vi "Run Command Gavin idk.vi"(2 "Line Index In":i32, 3 "Script":string) -> (0 "Line Index Out":i32, 1 "Done":bool)   [LabVIEW 2017, in "Apple script.lvlib"]
doc: "Looks at a line and runs the appropriate command. Add new commands to this vi."
uses:
  Apple script.lvlib
  Robot Global Data.vi
  <vilib>/addons/control/pid/pid.llb/PID.vi
  <vilib>/addons/control/pid/pid.llb/PID (DBL).vi
  Angle Distance.vi
  Pigeon Gyro.vi
  Encoders.vi
  Swerve Goto.vi
  <vilib>/Rock Robotics/Network Tables/NT Write Value.vi
  <vilib>/Rock Robotics/Network Tables/NT Write Numeric Array.vi
  Parse Number.vi
  Timer.vi
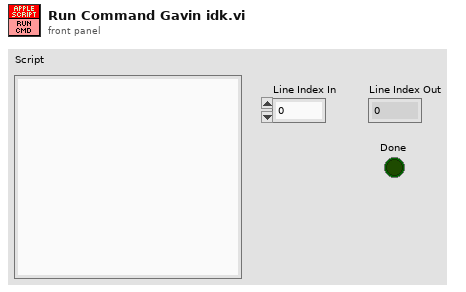
[diagram p1: front panel]
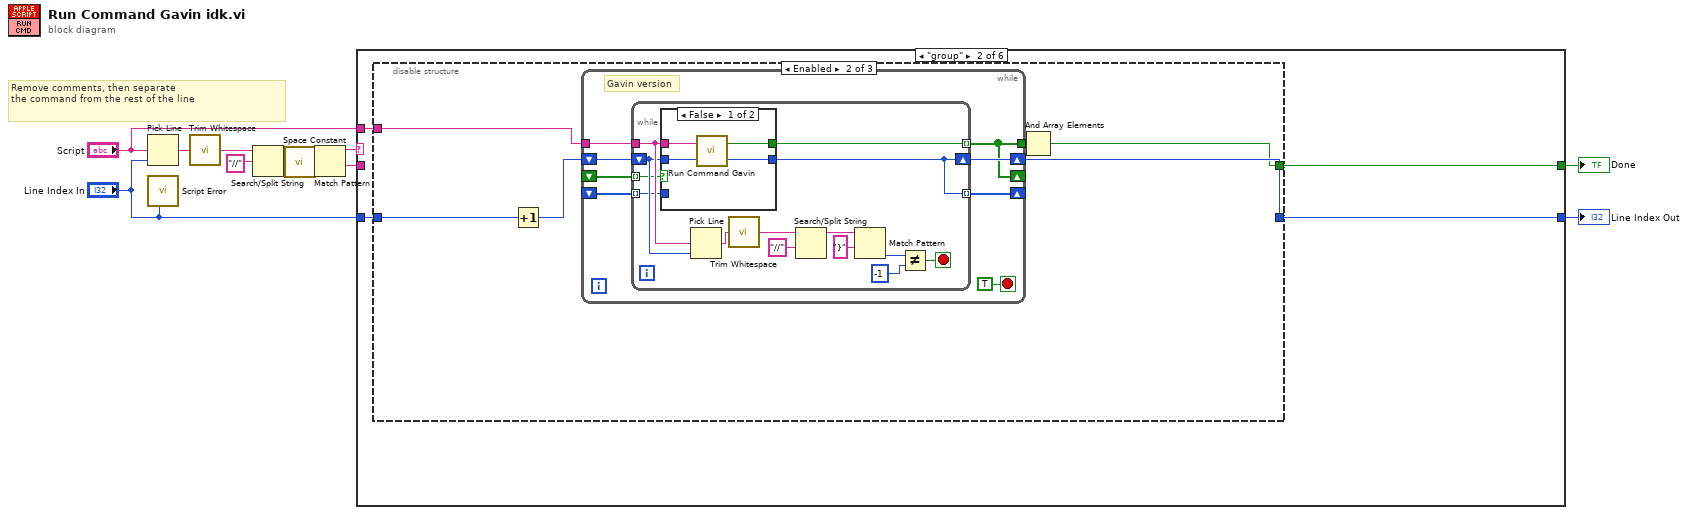
[diagram p0: block diagram]
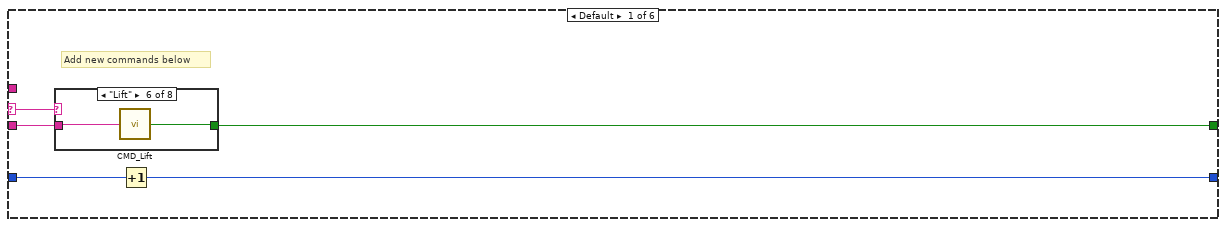
[diagram p2: hidden frame]
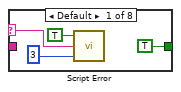
[diagram p3: hidden frame]
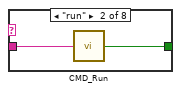
[diagram p4: hidden frame]
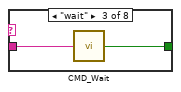
[diagram p5: hidden frame]
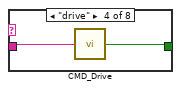
[diagram p6: hidden frame]
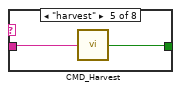
[diagram p7: hidden frame]
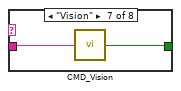
[diagram p8: hidden frame]
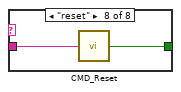
[diagram p9: hidden frame]
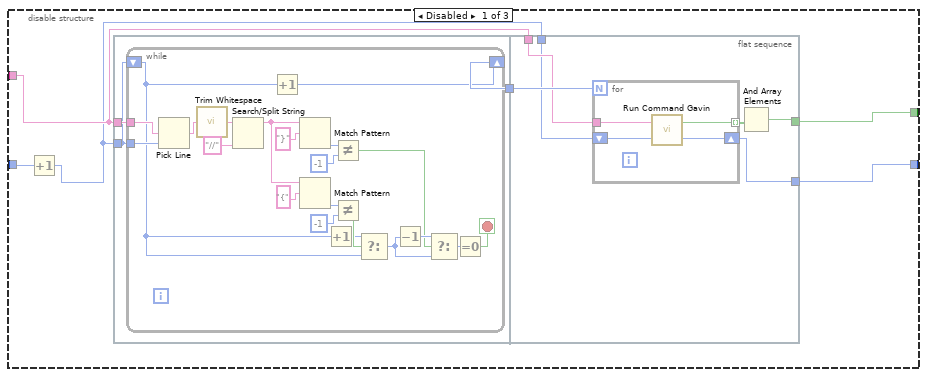
[diagram p10: hidden frame]
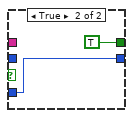
[diagram p11: hidden frame]
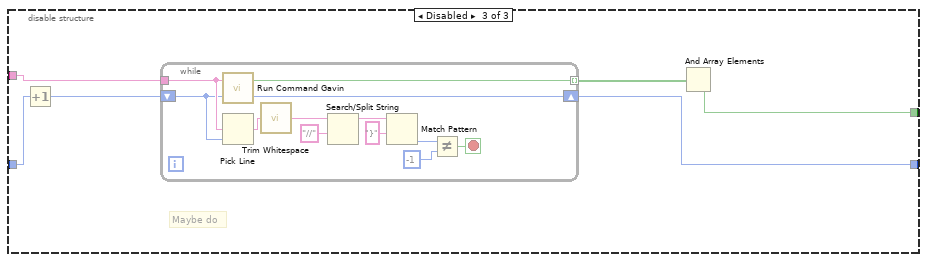
[diagram p12: hidden frame]
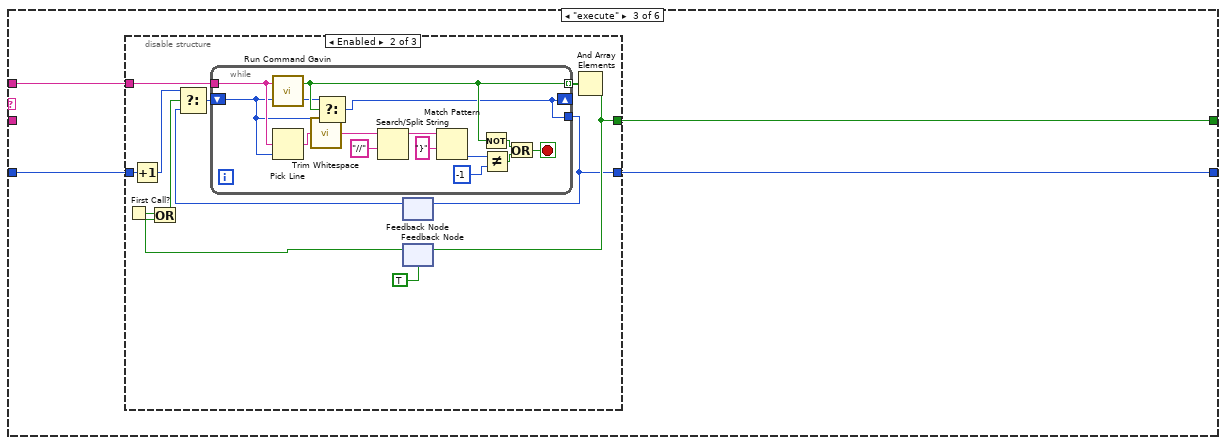
[diagram p13: hidden frame]
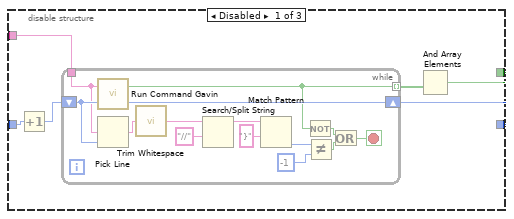
[diagram p14: hidden frame]
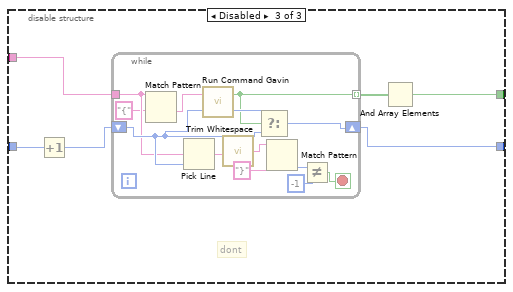
[diagram p15: hidden frame]
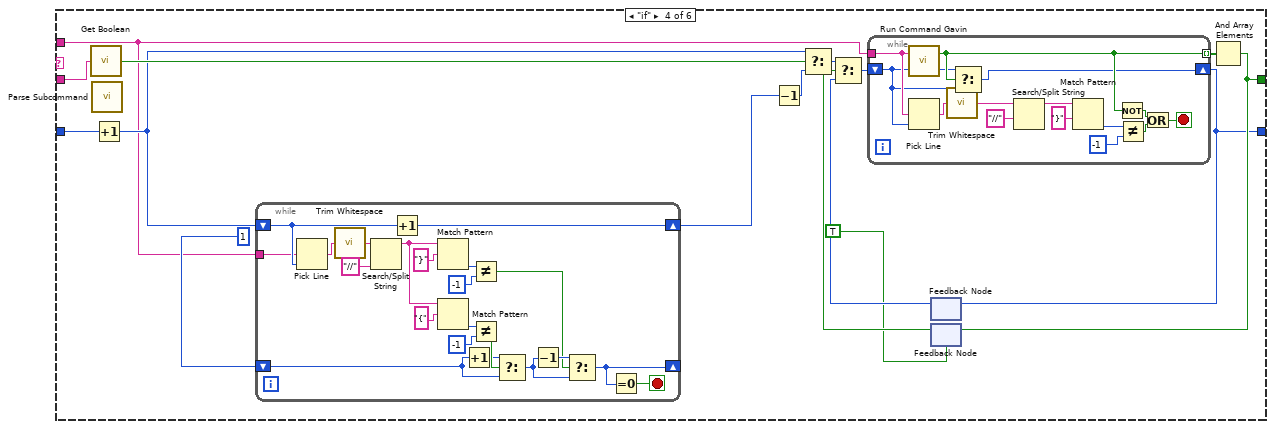
[diagram p16: hidden frame]
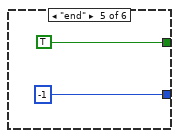
[diagram p17: hidden frame]
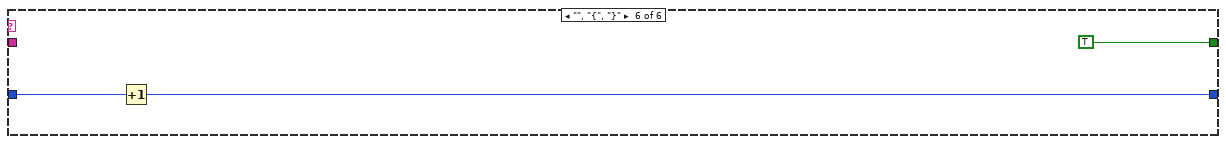
[diagram p18: hidden frame]
diagram:
  # "Remove comments, then separate\nthe command from the rest of the line"
  n1 = Pick Line(multi-line string="Script", line index="Line Index In") -> (output string=w8:string)  [unwired: 1 in]
  n2 = call "Script Error.vi"("Line Number"="Line Index In") -> ()  [unwired: 4 in, 1 out]
  n3 = call <vilib>:"Trim Whitespace.vi"("string"=w8) -> ("trimmed string"=w6:string)  [unwired: 1 in]
  n4 = Search/Split String(string=w6, search string/char (-)="//") -> (substring before match=w5:string)  [unwired: 1 in, 2 out]
  n5 = call <vilib>:"Space Constant.vi"() -> ("String"=w11:string)
  n6 = Match Pattern(string=w5, regular expression=w11) -> (before substring=w4:string, after substring=w3:string)  [unwired: 1 in, 2 out]
  n7 = case shown="\"group\"" w4 {
    selector: w4 -> [w14 _ _ _ _ _]
    tunnel: "Script" -> [_ w38 w131 w203 _ _]
    tunnel: "Line Index In" -> [w16 w36 w132 w215 _ w256]
    tunnel: [w13 w35 w134 w216 TRUE ("Running") TRUE ("Running")] -> w2
    tunnel: [w15 w37 w133 w213 -1 ("Line Index Out") w255] -> w1
    tunnel: w3 -> [w12 _ _ w214 _ _]
    frame Default {
      # "Add new commands below"
      n8 = case shown="\"Lift\"" w14 {
        selector: w14 -> [w17 _ _ _ _ _ _ _]
        tunnel: [TRUE w21 w24 w25 w27 w29 w31 w33] -> w13
        tunnel: w12 -> [_ w22 w23 w26 w28 w30 w32 w34]
        frame Default {
          n9 = call "Script Error.vi"("Error?"=TRUE, "Error Details"=w17, "Error Code"=3) -> ()  [unwired: 2 in, 1 out]
        }
        frame "run" {
          n10 = call "CMD_Run.vi"("Line"=w22) -> ("Done"=w21:bool)
        }
        frame "wait" {
          n11 = call "CMD_Wait.vi"("Line"=w23) -> ("Done"=w24:bool)
        }
        frame "drive" {
          n12 = call "CMD_Drive.vi"("Line"=w26) -> ("Done"=w25:bool)
        }
        frame "harvest" {
          n13 = call "CMD_Harvest.vi"("Line"=w28) -> ("Done"=w27:bool)
        }
        frame "Lift" {
          n14 = call "CMD_Lift.vi"("Line"=w30) -> ("Done"=w29:bool)
        }
        frame "Vision" {
          n15 = call "CMD_Vision.vi"("Line"=w32) -> ("Done"=w31:bool)
        }
        frame "reset" {
          n16 = call "CMD_Reset.vi"("Line"=w34) -> ("Done"=w33:bool)
        }
      }
      n17 = Increment(x=w16) -> (x+1=w15:i32)
    }
    frame "group" {
      n18 = disable-structure shown="Enabled" {
        disable-tunnel: w38 -> [w40 w82 w118]
        disable-tunnel: [w43 w80 w115] -> w37
        disable-tunnel: w36 -> [w42 w81 w117]
        disable-tunnel: [w44 w79 w113] -> w35
        frame Disabled {
          n19 = Increment(x=w42) -> (x+1=w39:i32)
          n20 = flat-sequence {
            tunnel: w40 -> [w46]
            tunnel: [w47] -> w41
            tunnel: w39 -> [w45]
            tunnel: [w74] -> w44
            tunnel: [w73] -> w43
            tunnel: w41 -> [w72]
            tunnel: w40 -> [w70]
            tunnel: w39 -> [w69]
            frame #0 {
              n21 = while {
                shift-right: [w68] -> w47
                shift-left: w45 -> [w48]
                tunnel: w46 -> [w51]
                tunnel: w45 -> [w50]
                stop <- w49 stop-if-true
                n22 = Pick Line(multi-line string=w51, line index=w50) -> (output string=w64:string)  [unwired: 1 in]
                n23 = call <vilib>:"Trim Whitespace.vi"("string"=w64) -> ("trimmed string"=w65:string)  [unwired: 1 in]
                n24 = Search/Split String(string=w65, search string/char (-)="//") -> (substring before match=w58:string)  [unwired: 1 in, 2 out]
                n25 = Increment(x=w48) -> (x+1=w68:i32)
                n26 = Match Pattern(string=w58, regular expression="}" ("search string/char (-)")) -> (offset past match=w67:i32)  [unwired: 1 in, 3 out]
                n27 = Match Pattern(string=w58, regular expression="{" ("search string/char (-)")) -> (offset past match=w59:i32)  [unwired: 1 in, 3 out]
                n28 = Increment(x=w48) -> (x+1=w56:i32)
                n29 = Not Equal?(x=w67, y=-1) -> (x != y?=w53:bool)
                n30 = Not Equal?(x=w59, y=-1) -> (x != y?=w57:bool)
                n31 = Select(t=w56, s=w57, f=w48) -> (s? t:f=w54:i32)
                n32 = Decrement(x=w54) -> (x-1=w55:i32)
                n33 = Select(t=w55, s=w53, f=w54) -> (s? t:f=w52:i32)
                n34 = Equal To 0?(x=w52) -> (x = 0?=w49:bool)
              }
            }
            frame #1 {
              n35 = for {
                N: w72 -> [_]
                tunnel: w70 -> [w78]
                tunnel: [w77] -> w71 mode=indexing
                shift-right: [w75] -> w73
                shift-left: w69 -> [w76]
                n36 = call "Run Command Gavin.vi"("Line Index In"=w76, "Script"=w78) -> ("Line Index Out"=w75:i32, "Done"=w77:bool)
              }
              n37 = And Array Elements(Boolean array=w71) -> (logical AND=w74:bool)
            }
          }
        }
        frame Enabled {
          n38 = Increment(x=w81) -> (x+1=w83:i32)
          n39 = while {
            tunnel: [w87] -> w84
            tunnel: w82 -> [w91]
            shift-right: [w90] -> w80
            shift-left: w83 -> [w92]
            shift-right: [w88] -> _
            shift-left: _ -> [w86]
            shift-right: [w87] -> _
            shift-left: _ -> [w85]
            stop <- TRUE stop-if-true
            # "Gavin version"
            n40 = while {
              tunnel: w91 -> [w106]
              tunnel: [w99] -> w87 mode=indexing
              shift-right: [w94] -> w90
              shift-left: w92 -> [w98]
              tunnel: w85 -> [w95] mode=indexing
              tunnel: [w94] -> w88 mode=indexing
              tunnel: w86 -> [w93] mode=indexing
              stop <- w96 stop-if-true
              n41 = case shown="False" w95 {
                tunnel: w106 -> [w110 _]
                tunnel: [w107 TRUE ("Done")] -> w99
                tunnel: w98 -> [w109 _]
                tunnel: [w108 w111] -> w94
                tunnel: w93 -> [_ w111]
                frame False {
                  n42 = call "Run Command Gavin.vi"("Line Index In"=w109, "Script"=w110) -> ("Line Index Out"=w108:i32, "Done"=w107:bool)
                }
                frame True {
                }
              }
              n43 = Pick Line(multi-line string=w106, line index=w98) -> (output string=w101:string)  [unwired: 1 in]
              n44 = call <vilib>:"Trim Whitespace.vi"("string"=w101) -> ("trimmed string"=w102:string)  [unwired: 1 in]
              n45 = Search/Split String(string=w102, search string/char (-)="//") -> (substring before match=w97:string)  [unwired: 1 in, 2 out]
              n46 = Match Pattern(string=w97, regular expression="}" ("search string/char (-)")) -> (offset past match=w104:i32)  [unwired: 1 in, 3 out]
              n47 = Not Equal?(x=w104, y=-1) -> (x != y?=w96:bool)
            }
          }
          n48 = And Array Elements(Boolean array=w84) -> (logical AND=w79:bool)
        }
        frame Disabled {
          # "Maybe do"
          n49 = Increment(x=w117) -> (x+1=w116:i32)
          n50 = while {
            tunnel: w118 -> [w130]
            tunnel: [w123] -> w114 mode=indexing
            shift-right: [w120] -> w115
            shift-left: w116 -> [w122]
            stop <- w121 stop-if-true
            n51 = call "Run Command Gavin.vi"("Line Index In"=w122, "Script"=w130) -> ("Line Index Out"=w120:i32, "Done"=w123:bool)
            n52 = Pick Line(multi-line string=w130, line index=w122) -> (output string=w125:string)  [unwired: 1 in]
            n53 = call <vilib>:"Trim Whitespace.vi"("string"=w125) -> ("trimmed string"=w126:string)  [unwired: 1 in]
            n54 = Search/Split String(string=w126, search string/char (-)="//") -> (substring before match=w119:string)  [unwired: 1 in, 2 out]
            n55 = Match Pattern(string=w119, regular expression="}" ("search string/char (-)")) -> (offset past match=w128:i32)  [unwired: 1 in, 3 out]
            n56 = Not Equal?(x=w128, y=-1) -> (x != y?=w121:bool)
          }
          n57 = And Array Elements(Boolean array=w114) -> (logical AND=w113:bool)
        }
      }
    }
    frame "execute" {
      n58 = disable-structure shown="Enabled" {
        disable-tunnel: [w137 w159 w183] -> w134
        disable-tunnel: [w138 w155 w182] -> w133
        disable-tunnel: w132 -> [w136 w166 w186]
        disable-tunnel: w131 -> [w139 w164 w187]
        frame Disabled {
          n59 = Increment(x=w136) -> (x+1=w135:i32)
          n60 = while {
            tunnel: w139 -> [w146]
            tunnel: [w142] -> w140 mode=indexing
            shift-right: [w154] -> w138
            shift-left: w135 -> [w147]
            stop <- w145 stop-if-true
            n61 = call "Run Command Gavin.vi"("Line Index In"=w147, "Script"=w146) -> ("Line Index Out"=w154:i32, "Done"=w142:bool)
            n62 = Pick Line(multi-line string=w146, line index=w147) -> (output string=w149:string)  [unwired: 1 in]
            n63 = call <vilib>:"Trim Whitespace.vi"("string"=w149) -> ("trimmed string"=w150:string)  [unwired: 1 in]
            n64 = Search/Split String(string=w150, search string/char (-)="//") -> (substring before match=w141:string)  [unwired: 1 in, 2 out]
            n65 = Match Pattern(string=w141, regular expression="}" ("search string/char (-)")) -> (offset past match=w152:i32)  [unwired: 1 in, 3 out]
            n66 = Not(x=w142) -> (.not. x?=w143:bool)
            n67 = Not Equal?(x=w152, y=-1) -> (x != y?=w144:bool)
            n68 = Or(x=w143, y=w144) -> (x .or. y?=w145:bool)
          }
          n69 = And Array Elements(Boolean array=w140) -> (logical AND=w137:bool)
        }
        frame Enabled {
          n70 = First Call?() -> (First Call?: T/F=w156:bool)
          n71 = Increment(x=w166) -> (x+1=w162:i32)
          n72 = feedback #1() -> (w161:i32)  [unwired: 1 in]
          n73 = feedback #2(TRUE) -> (w160:bool)
          n74 = Or(x=w156, y=w160) -> (x .or. y?=w157:bool)
          n75 = Select(t=w162, s=w157, f=w161) -> (s? t:f=w163:i32)
          n76 = while {
            tunnel: w164 -> [w181]
            tunnel: [w171] -> w165 mode=indexing
            shift-right: [w167] -> _
            shift-left: w163 -> [w169]
            tunnel: [w167] -> w155
            stop <- w180 stop-if-true
            n77 = call "Run Command Gavin.vi"("Line Index In"=w169, "Script"=w181) -> ("Line Index Out"=w170:i32, "Done"=w171:bool)
            n78 = Pick Line(multi-line string=w181, line index=w169) -> (output string=w175:string)  [unwired: 1 in]
            n79 = call <vilib>:"Trim Whitespace.vi"("string"=w175) -> ("trimmed string"=w176:string)  [unwired: 1 in]
            n80 = Select(t=w170, s=w171, f=w169) -> (s? t:f=w167:i32)
            n81 = Search/Split String(string=w176, search string/char (-)="//") -> (substring before match=w168:string)  [unwired: 1 in, 2 out]
            n82 = Match Pattern(string=w168, regular expression="}" ("search string/char (-)")) -> (offset past match=w178:i32)  [unwired: 1 in, 3 out]
            n83 = Not(x=w171) -> (.not. x?=w172:bool)
            n84 = Not Equal?(x=w178, y=-1) -> (x != y?=w173:bool)
            n85 = Or(x=w172, y=w173) -> (x .or. y?=w180:bool)
          }
          n86 = feedback-in #1(w155) -> ()
          n87 = And Array Elements(Boolean array=w165) -> (logical AND=w159:bool)
          n88 = feedback-in #2(w159) -> ()
        }
        frame Disabled {
          # "dont"
          n89 = Increment(x=w186) -> (x+1=w185:i32)
          n90 = while {
            tunnel: w187 -> [w190]
            tunnel: [w199] -> w184 mode=indexing
            shift-right: [w198] -> w182
            shift-left: w185 -> [w191]
            stop <- w192 stop-if-true
            n91 = Match Pattern(string=w190, regular expression="{") -> (after substring=w188:string)  [unwired: 1 in, 3 out]
            n92 = Pick Line(multi-line string=w190, line index=w191) -> (output string=w197:string)  [unwired: 1 in]
            n93 = call "Run Command Gavin.vi"("Line Index In"=w191, "Script"=w188) -> ("Line Index Out"=w200:i32, "Done"=w199:bool)
            n94 = call <vilib>:"Trim Whitespace.vi"("string"=w197) -> ("trimmed string"=w196:string)  [unwired: 1 in]
            n95 = Select(t=w200, s=w199, f=w191) -> (s? t:f=w198:i32)
            n96 = Match Pattern(string=w196, regular expression="}") -> (offset past match=w194:i32)  [unwired: 1 in, 3 out]
            n97 = Not Equal?(x=w194, y=-1) -> (x != y?=w192:bool)
          }
          n98 = And Array Elements(Boolean array=w184) -> (logical AND=w183:bool)
        }
      }
    }
    frame "if" {
      n99 = call "Get Boolean.vi"("Name"=w214) -> ("Value"=w207:bool)
      n100 = call "Parse Subcommand.vi"() -> ()  [unwired: 9 in, 7 out]
      n101 = Increment(x=w215) -> (x+1=w205:i32)
      n102 = while {
        shift-right: [w230] -> w204
        shift-left: w205 -> [w232]
        shift-right: [w218] -> _
        shift-left: 1 -> [w223]
        tunnel: w203 -> [w217]
        stop <- w219 stop-if-true
        n103 = Pick Line(multi-line string=w217, line index=w232) -> (output string=w234:string)  [unwired: 1 in]
        n104 = call <vilib>:"Trim Whitespace.vi"("string"=w234) -> ("trimmed string"=w235:string)  [unwired: 1 in]
        n105 = Search/Split String(string=w235, search string/char (-)="//") -> (substring before match=w226:string)  [unwired: 1 in, 2 out]
        n106 = Increment(x=w232) -> (x+1=w230:i32)
        n107 = Match Pattern(string=w226, regular expression="}" ("search string/char (-)")) -> (offset past match=w237:i32)  [unwired: 1 in, 3 out]
        n108 = Match Pattern(string=w226, regular expression="{" ("search string/char (-)")) -> (offset past match=w227:i32)  [unwired: 1 in, 3 out]
        n109 = Increment(x=w223) -> (x+1=w224:i32)
        n110 = Not Equal?(x=w237, y=-1) -> (x != y?=w220:bool)
        n111 = Not Equal?(x=w227, y=-1) -> (x != y?=w225:bool)
        n112 = Select(t=w224, s=w225, f=w223) -> (s? t:f=w221:i32)
        n113 = Decrement(x=w221) -> (x-1=w222:i32)
        n114 = Select(t=w222, s=w220, f=w221) -> (s? t:f=w218:i32)
        n115 = Equal To 0?(x=w218) -> (x = 0?=w219:bool)
      }
      n116 = Decrement(x=w204) -> (x-1=w201:i32)
      n117 = Select(t=w205, s=w207, f=w201) -> (s? t:f=w208:i32)
      n118 = feedback #3() -> (w209:i32)  [unwired: 1 in]
      n119 = feedback #4(TRUE) -> (w212:bool)
      n120 = Select(t=w208, s=w212, f=w209) -> (s? t:f=w211:i32)
      n121 = while {
        tunnel: w203 -> [w252]
        tunnel: [w242] -> w210 mode=indexing
        shift-right: [w239] -> w213
        shift-left: w211 -> [w240]
        stop <- w251 stop-if-true
        n122 = call "Run Command Gavin.vi"("Line Index In"=w240, "Script"=w252) -> ("Line Index Out"=w241:i32, "Done"=w242:bool)
        n123 = Pick Line(multi-line string=w252, line index=w240) -> (output string=w246:string)  [unwired: 1 in]
        n124 = call <vilib>:"Trim Whitespace.vi"("string"=w246) -> ("trimmed string"=w247:string)  [unwired: 1 in]
        n125 = Select(t=w241, s=w242, f=w240) -> (s? t:f=w239:i32)
        n126 = Search/Split String(string=w247, search string/char (-)="//") -> (substring before match=w238:string)  [unwired: 1 in, 2 out]
        n127 = Match Pattern(string=w238, regular expression="}" ("search string/char (-)")) -> (offset past match=w249:i32)  [unwired: 1 in, 3 out]
        n128 = Not(x=w242) -> (.not. x?=w243:bool)
        n129 = Not Equal?(x=w249, y=-1) -> (x != y?=w244:bool)
        n130 = Or(x=w243, y=w244) -> (x .or. y?=w251:bool)
      }
      n131 = feedback-in #3(w213) -> ()
      n132 = And Array Elements(Boolean array=w210) -> (logical AND=w216:bool)
      n133 = feedback-in #4(w216) -> ()
    }
    frame "end" {
    }
    frame "", "{", "}" {
      n134 = Increment(x=w256) -> (x+1=w255:i32)
    }
  }
  "Line Index Out" <- w1
  "Done" <- w2
